vi "7270 no valid cell at row column-error--error.vi"(8 "error in":errorcluster, 10 "Col":i32, 11 "Row":i32) -> (0 "error out":errorcluster)   [LabVIEW 2023, in "SourceGrid.lvlib" / "SourceGrid.lvclass"]
uses:
  SourceGrid.lvclass
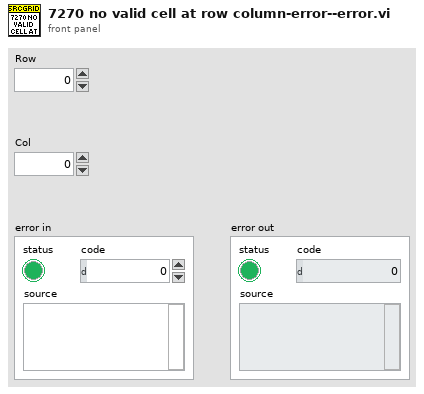
[diagram p1: front panel]
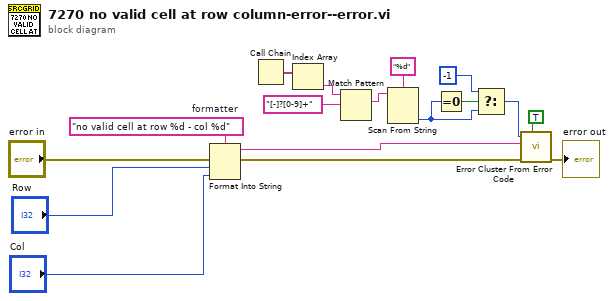
[diagram p0: block diagram]
diagram:
  w14 = "no valid cell at row %d - col %d"  # formatter
  n1 = Format Into String(format string=w14, error in="error in", "Row", "Col") -> (resulting string=w15:string, error out=w3:errorcluster)  [unwired: 1 in]
  n2 = Call Chain() -> (call chain=w5:string[])
  n3 = Index Array(array=w5) -> (element=w10:string)  [unwired: 1 in]
  n4 = Match Pattern(string=w10, regular expression="[-]?[0-9]+") -> (match substring=w11:string)  [unwired: 1 in, 3 out]
  n5 = Scan From String(format string="%d", input string=w11) -> (output 1=w7:i32)  [unwired: 3 in, 3 out]
  n6 = Equal To 0?(x=w7) -> (x = 0?=w8:bool)
  n7 = Select(t=-1, s=w8, f=w7) -> (s? t:f=w1:i32)
  n8 = call <vilib>:"Error Cluster From Error Code.vi"("show call chain? (False)"=TRUE, "error in (no error)"=w3, "error message (\"\")"=w15, "error code (0)"=w1) -> ("error out"=→"error out":errorcluster)  [unwired: 5 in]
